vi "example 3 - subpanel.vi"() -> ()   [LabVIEW 2020]
uses:
  ui-testing/ui-testing.lvlib
panel:
  in  "sub2":bool
  in  "sub1":bool
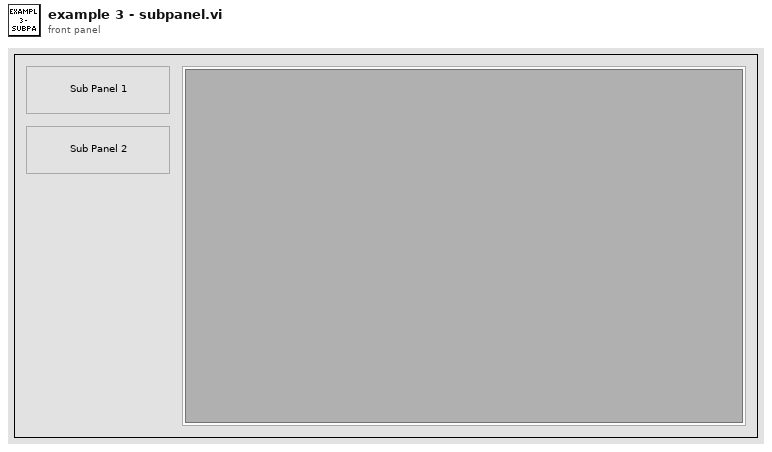
[diagram p1: front panel]
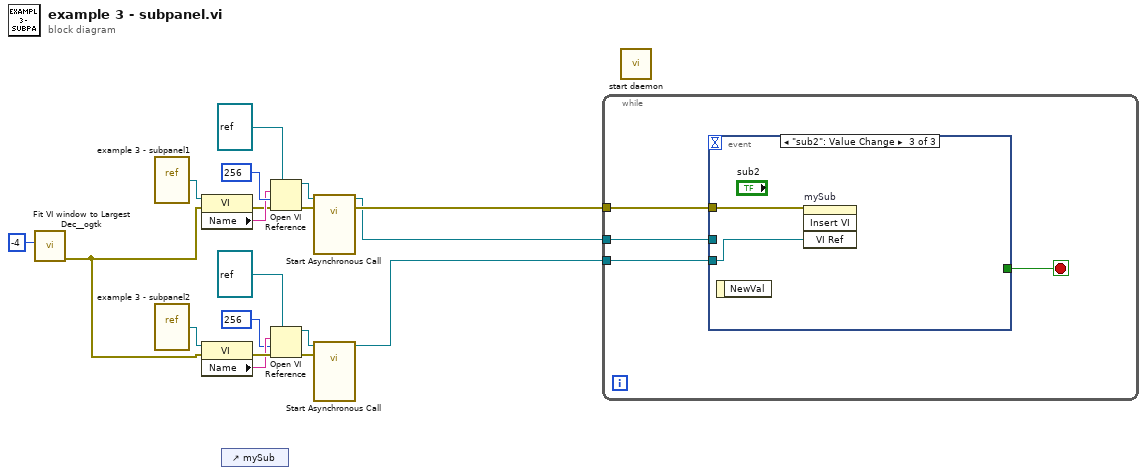
[diagram p0: block diagram]
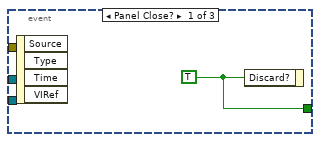
[diagram p2: hidden frame]
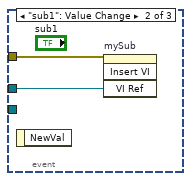
[diagram p3: hidden frame]
diagram:
  n1 = call <userlib>:"Fit VI window to Largest Dec__ogtk.vi"("border spacing (2 px)"=-4) -> ("error out"=w1:errorcluster)  [unwired: 5 in, 1 out]
  n2 = vi-ref "example 3 - subpanel1.vi"() -> (w15:refnum<vi>)
  n3 = vi-ref "example 3 - subpanel2.vi"() -> (w8:refnum<vi>)
  n4 = property class="VI"(reference=w15, error in=w1) -> (error out=w13:errorcluster, "Name"=w14:string)  [unwired: 1 out]
  n5 = property class="VI"(reference=w8, error in=w1) -> (error out=w10:errorcluster, "Name"=w9:string)  [unwired: 1 out]
  n6 = control-ref of="mySub"() -> ()  [unwired: 1 out]
  n7 = Open VI Reference(type specifier VI Refnum (for type only)=refnum<vi> refnum, vi path=w14, options=256 ("call and forget"), error in (no error)=w13) -> (vi reference=w17:refnum<vi>, error out=w16:errorcluster)  [unwired: 2 in]
  n8 = Open VI Reference(type specifier VI Refnum (for type only)=refnum<vi> refnum, vi path=w9, options=256 ("call and forget"), error in (no error)=w10) -> (vi reference=w6:refnum<vi>, error out=w7:errorcluster)  [unwired: 2 in]
  n9 = call-by-ref "Start Asynchronous Call"(reference=w17, error in=w16) -> (reference out=w11:refnum<vi>, error out=w12:errorcluster)  [unwired: 12 in]
  n10 = call-by-ref "Start Asynchronous Call"(reference=w6, error in=w7) -> (reference out=w3:refnum<vi>)  [unwired: 12 in, 1 out]
  n11 = while {
    tunnel: w12 -> [w22]
    tunnel: w11 -> [w21]
    tunnel: w3 -> [w20]
    stop <- w23 stop-if-true
    n12 = event shown="[2] \"sub2\": Value Change" {
      selector: _ -> [_ _ _]
      dyn-events: _ -> [_ _ _]
      timeout: _ -> [_ _ _]
      tunnel: [w24 _ _] -> w23
      tunnel: w22 -> [_ w26 w28]
      tunnel: w21 -> [_ w25 _]
      tunnel: w20 -> [_ _ w27]
      event Panel Close? {
        w24 = TRUE
        n13 = event-data() -> ()  [unwired: 1 in, 4 out]
        n14 = event-data("Discard?"=w24) -> ()  [unwired: 1 in, 1 out]
      }
      event "sub1": Value Change {
        n15 = event-data() -> ()  [unwired: 1 in, 1 out]
        n16 = invoke on="mySub" class="SubPnl" method="Insert VI"(error in=w26, "VI Ref"=w25) -> ()  [unwired: 2 in, 4 out]
      }
      event "sub2": Value Change {
        n17 = event-data() -> ()  [unwired: 1 in, 1 out]
        n18 = invoke on="mySub" class="SubPnl" method="Insert VI"(error in=w28, "VI Ref"=w27) -> ()  [unwired: 2 in, 4 out]
      }
    }
  }
  n19 = call "start daemon.vi"() -> ()  [unwired: 11 in, 1 out]
